vi "Power Qualtiy - 3.vi"() -> ()   [LabVIEW 2015]
uses:
  <vilib>/express/express analysis/Spectral/Block/exnSpectralBlock spectral measurements RMS poly.vi
  <vilib>/express/express analysis/Spectral/Block/exnSpectralBlock spectral measurements RMS DDT.vi
  <vilib>/express/express analysis/Spectral/XNode/ExpressSpectralMeasurementsBlockNode.xnode
panel:
  out "Power":dbl
  out "Peak to Peak 2":dbl
  out "Current Harmonics":dynamicdata(graph)
  out "Voltage Harmonics":dynamicdata(graph)
  out "current":dbl
  out "voltage":dbl
  out "current Graph":dynamicdata(graph)
  out "voltage Graph":dynamicdata(graph)
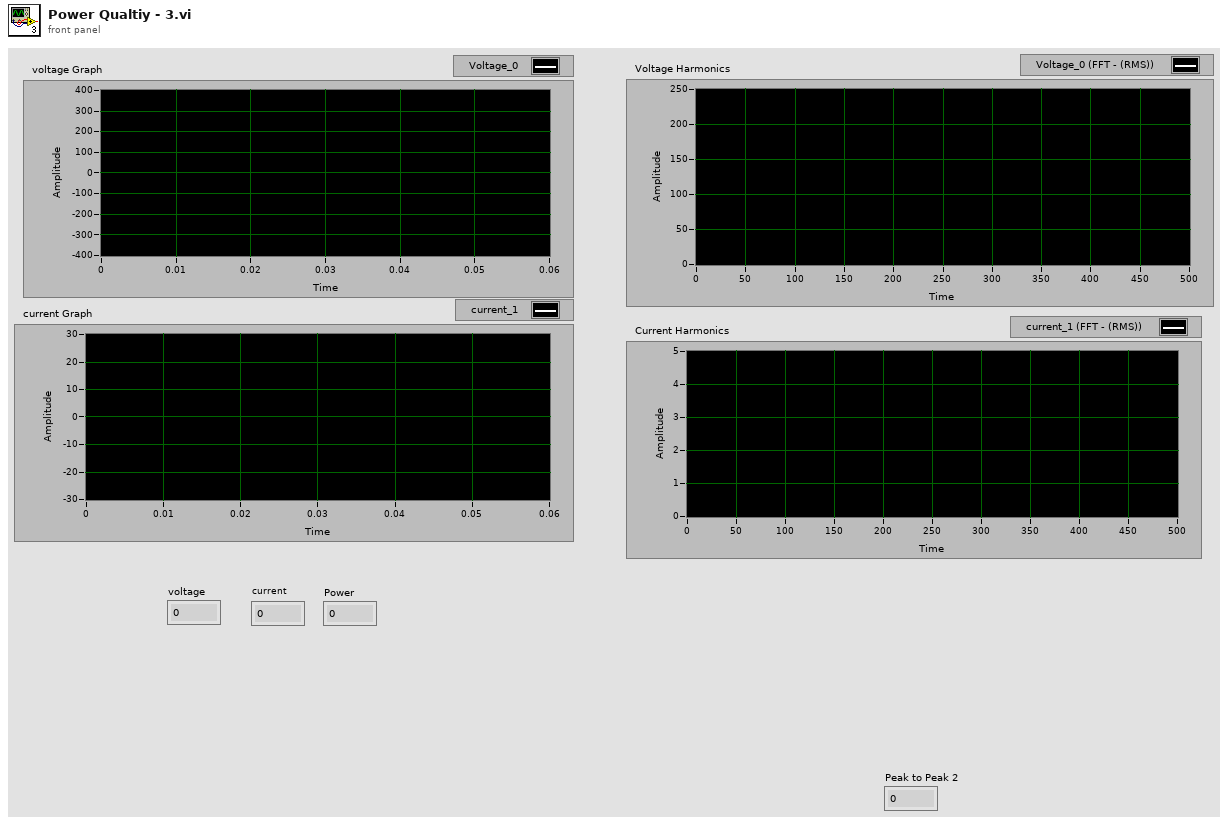
[diagram p1: front panel]
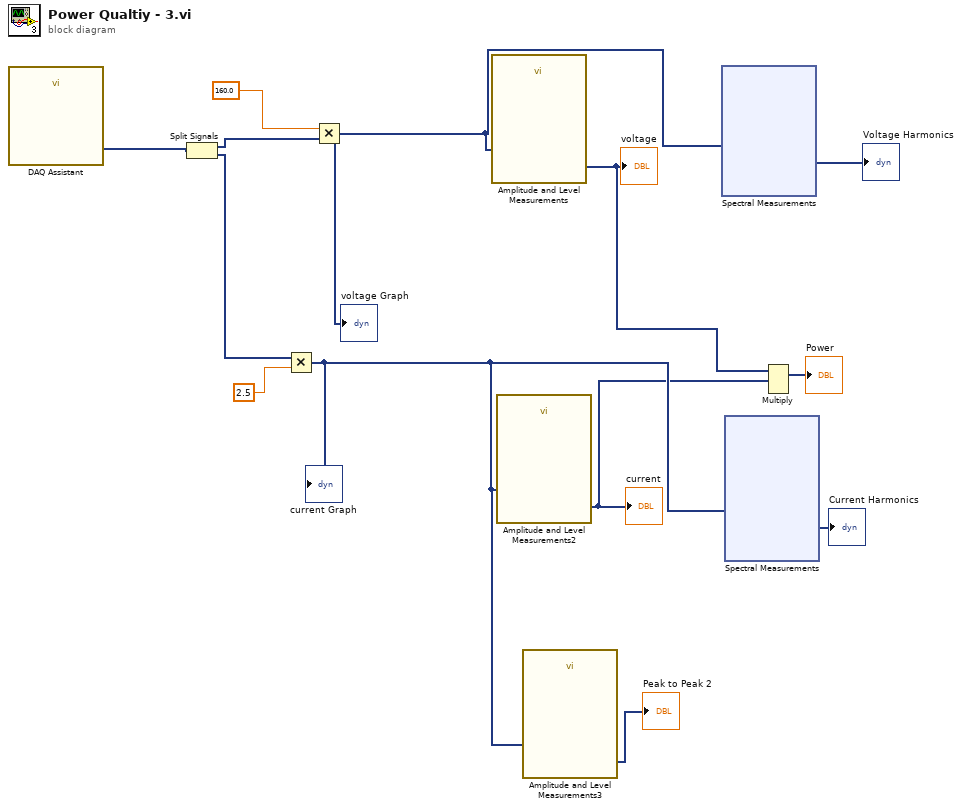
[diagram p0: block diagram]
diagram:
  n1 = call "DAQ Assistant"() -> ("data"=w1:dynamicdata)  [unwired: 16 in, 3 out]
  n2 = Split Signals(w1) -> (w12:dynamicdata, w10:dynamicdata)  [unwired: 2 in]
  n3 = Multiply(x=w10, y=2.5) -> (x*y=w6:dynamicdata)
  "current Graph" <- w6
  n4 = Multiply(x=160.0, y=w12) -> (x*y=w9:dynamicdata)
  "voltage Graph" <- w9
  n5 = call "Amplitude and Level Measurements"("Signals"=w9) -> ("RMS"=w4:dynamicdata)  [unwired: 13 in, 1 out]
  "voltage" <- w4
  n6 = call "Amplitude and Level Measurements2"("Signals"=w6) -> ("RMS"=w3:dynamicdata)  [unwired: 13 in, 1 out]
  "current" <- w3
  n7 = call "Amplitude and Level Measurements3"("Signals"=w6) -> ("Peak to Peak"=→"Peak to Peak 2":dynamicdata)  [unwired: 13 in, 1 out]
  n8 = xnode "Spectral Measurements"("Signals"=w9) -> ("FFT - (RMS)"=→"Voltage Harmonics":dynamicdata)  [unwired: 1 in, 2 out]
  n9 = xnode "Spectral Measurements"("Signals"=w6) -> ("FFT - (RMS)"=→"Current Harmonics":dynamicdata)  [unwired: 1 in, 2 out]
  n10 = Multiply(1:w3, 2:w4) -> (0:→"Power":dynamicdata)  [unwired: 1 in, 1 out]
